vi "Polling Core.vi"(8 "Error In":errorcluster, 11 "CS++IEFWerner in":refnum<class "CS++IEFWerner.lvclass">) -> (0 "Error Out":errorcluster, 3 "CS++IEFWerner out":refnum<class "CS++IEFWerner.lvclass">)   [LabVIEW 2015, in "CS++IEFWerner.lvlib" / "CS++IEFWerner.lvclass"]
doc: "Implement the pseudo-periodic action in your override.vi."
uses:
  CS++IEFWerner.lvclass
  CSPP_Core/Actors/CS++BaseActor/CS++BaseActor.lvclass/CS++BaseActor.ctl
  CSPP_Core/Actors/CS++BaseActor/CS++BaseActor.lvclass
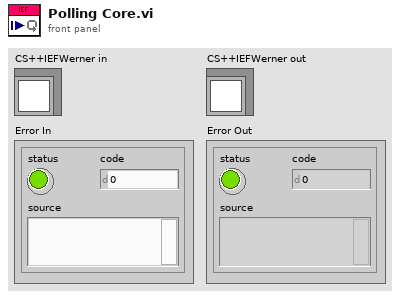
[diagram p1: front panel]
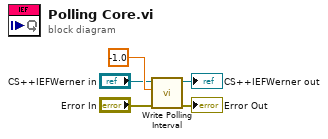
[diagram p0: block diagram]
diagram:
  n1 = call "Write Polling Interval.vi"("error in (no error)"="Error In", "Polling Interval"=dbl[unit] -1.0, "CS++BaseActor in"="CS++IEFWerner in") -> ("error out"=→"Error Out":errorcluster, "CS++BaseActor out"=→"CS++IEFWerner out":refnum<class "CS++IEFWerner.lvclass">)  [unwired: 7 in]
